vi "Sync_Correlation_low.vi"(0 "Shift In":dbl[](array[numeric]) format="%.2f", 1 "Analogue Data":dbl[](array[numeric]) format="%.2f", 2 "Block No":i32=1, 5 "Delay (ms)":dbl format="%.2f", 9 "Arrival Times":dbl[](array[numeric]) format="%.2f", 11 "Delta T (ms)":dbl format="%.2f", 12 "T":dbl[](array[numeric]) format="%.2f", 13 "U":dbl[](array[numeric]) format="%.2f", 14 "W":dbl[](array[numeric]) format="%.2f") -> (4 "Shift Out":dbl[](array[numeric]) format="%.2f")   [LabVIEW 2010]
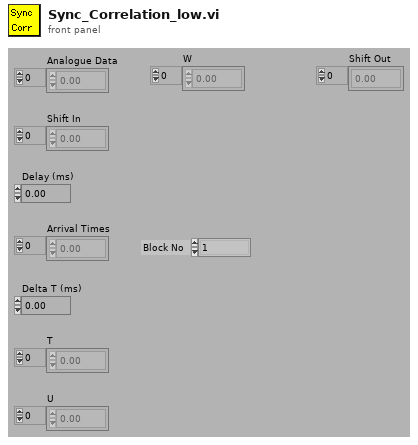
[diagram p1: front panel]
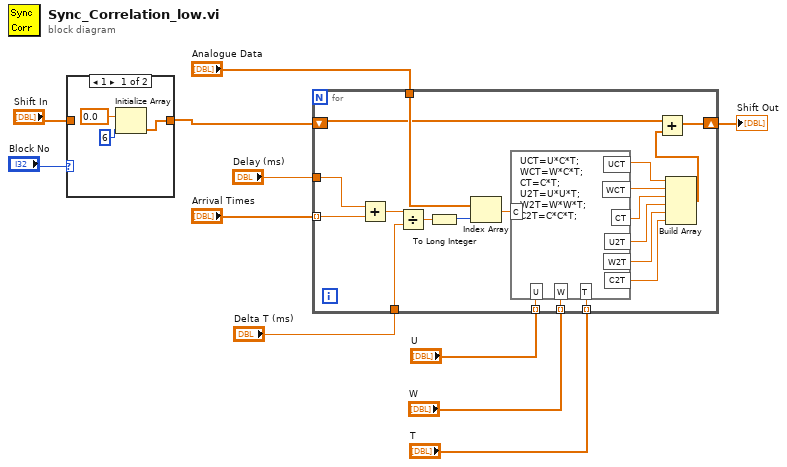
[diagram p0: block diagram]
diagram:
  n1 = case shown="1" "Block No" {
    tunnel: [w12 w15] -> w2
    tunnel: "Shift In" -> [_ w15]
    frame 1 {
      n2 = Initialize Array(0.0 ("Element Data"), 6 ("Dimension Size")) -> (w12:dbl[])
    }
    frame 2, Default {
    }
  }
  n3 = for {
    tunnel: "Arrival Times" -> [w35] mode=indexing
    tunnel: "Delay (ms)" -> [w34]
    tunnel: "Delta T (ms)" -> [w32]
    tunnel: "Analogue Data" -> [w29]
    tunnel: "U" -> [w28] mode=indexing
    tunnel: "W" -> [w27] mode=indexing
    tunnel: "T" -> [w26] mode=indexing
    shift-right: [w20] -> w11
    shift-left: w2 -> [w19]
    n4 = Add(x=w34, y=w35) -> (x+y=w33:dbl)
    n5 = Divide(x=w33, y=w32) -> (x/y=w31:dbl)
    n6 = To Long Integer(number=w31) -> (32bit integer=w30:i32)
    n7 = Index Array(array=w29, index=w30) -> (element=w25:dbl)
    n8 = formula code="UCT=U*C*T;\nWCT=W*C*T;\nCT=C*T;\nU2T=U*U*T;\nW2T=W*W*T;\nC2T=C*C*T;"("W"=w27, "U"=w28, "T"=w26, "C"=w25) -> ("UCT"=w24:dbl, "WCT"=w23:dbl, "CT"=w22:dbl, "U2T"=w18:dbl, "W2T"=w17:dbl, "C2T"=w16:dbl)
    n9 = Build Array(w24, w23, w22, w18, w17, w16) -> (w21:dbl[])
    n10 = Add(x=w19, y=w21) -> (x+y=w20:dbl[])
  }
  "Shift Out" <- w11
